vi "Point_Read_All.vi"(8 "Error In":errorcluster, 11 "Map":T3) -> (0 "Error Out":errorcluster, 1 "Points":T1[](array[typedef]), 2 "Names":string[](array[string]), 3 "Map Out":T3)   [LabVIEW 2017, in "PointValueMap.lvlib"]
doc: "Reads out all of the points stored in the map in their raw format."
uses:
  <vilib>/addons/PointValueMap/PointValueMap.lvlib
  <vilib>/addons/PointValueMap/controls/PointMap.ctl
  <vilib>/addons/PointValueMap/controls/Point.ctl
  <vilib>/addons/PointValueMap/controls/DataTypes.ctl
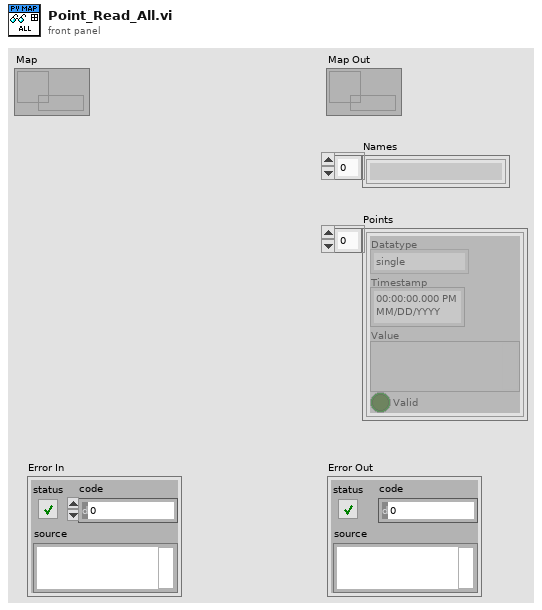
[diagram p1: front panel]
types:
  T1 = typedef "PointValueMap.lvlib/Point.ctl" = cluster{"Datatype":T2, "Timestamp":timestamp, "Value":variant, "Valid":bool}
  T2 = typedef "PointValueMap.lvlib/DataTypes.ctl" = enum16{"single", "double", "i32", "string", "variant"}
  T3 = typedef "PointValueMap.lvlib/PointMap.ctl" = refnum<data-value>
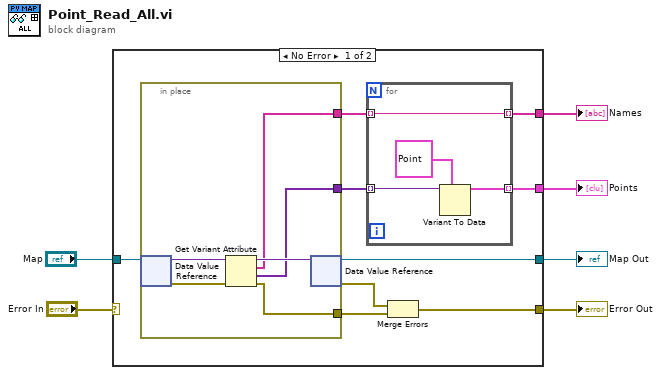
[diagram p0: block diagram]
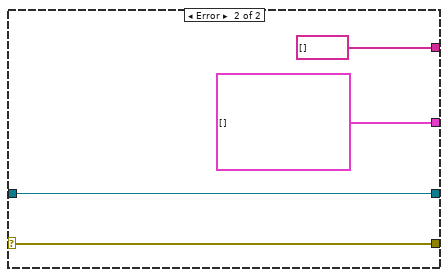
[diagram p2: hidden frame]
diagram:
  n1 = case shown="No Error" "Error In" {
    selector: "Error In" -> [_ w29]
    tunnel: "Map" -> [w15 w28]
    tunnel: [w13 w29] -> w6
    tunnel: [w11 w28] -> w3
    tunnel: [w8 string[] []] -> w2
    tunnel: [w7 T1[] []] -> w1
    frame No Error {
      n2 = in-place {
        in-place-border: [w22] -> w12
        in-place-border: [w20] -> w10
        in-place-border: [w21] -> w9
        n3 = in-place-dvr #1(w15) -> (w25:variant, w24:errorcluster)
        n4 = Get Variant Attribute(Variant=w25, error in=w24) -> (duplicate Variant=w23:variant, names=w20:string[], values=w21:variant[], error out=w22:errorcluster)  [unwired: 2 in]
        n5 = in-place-dvr #1(w23) -> (w11:T3, w14:errorcluster)
      }
      n6 = for {
        tunnel: w10 -> [w17] mode=indexing
        tunnel: w9 -> [w19] mode=indexing
        tunnel: [w17] -> w8 mode=indexing
        tunnel: [w16] -> w7 mode=indexing
        n7 = Variant To Data(type=T1 {"Datatype"=enum."single", "Timestamp"=timestamp(0 s since 1904-01-01), "Value"=variant, "Valid"=FALSE} ("Point"), Variant=w19) -> (data=w16:T1)  [unwired: 1 in, 1 out]
      }
      n8 = Merge Errors(w14, w12) -> (w13:errorcluster)
    }
    frame Error {
    }
  }
  "Error Out" <- w6
  "Names" <- w2
  "Map Out" <- w3
  "Points" <- w1
